vi "ReadINI.vi"(8 "error in (no error)":errorcluster) -> (0 "error out":errorcluster, 2 "FileNotFound/Corrupted?":bool, 3 "value":T1={"ClientTimeout (s)"=30, "LogPath"=path "", "CriticalErrors"=[], "OracleData"={"DBname"="", "User"="", "Password"=""}})   [LabVIEW 2017, in "Server.lvlib"]
doc: "Reads the INI-File and decodes the XML-String to ServerINI.ctl-Cluster. If File not found or File content doesnt fit to the ctl it outputs a bool."
uses:
  Server.lvlib
  TypeDefs/ServerINI.ctl
  SubLibs/Oracle/OracleData.ctl
  SubLibs/Oracle/Oracle.lvlib
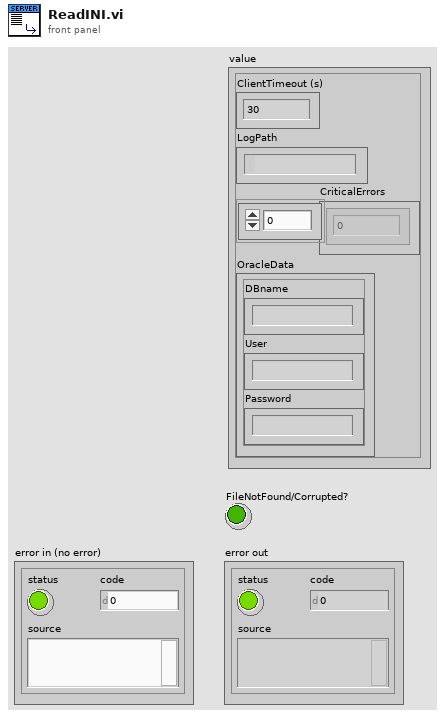
[diagram p1: front panel]
types:
  T1 = typedef "Server.lvlib/ServerINI.ctl" = cluster{"ClientTimeout (s)":u32, "LogPath":path, "CriticalErrors":i32[], "OracleData":T2}
  T2 = typedef "Server.lvlib/Oracle.lvlib/OracleData.ctl" = cluster{"DBname":string, "User":string, "Password":string}
  T3 = enum16{"open", "replace", "create", "open or create", "replace or create", "replace or create with confirmation"}
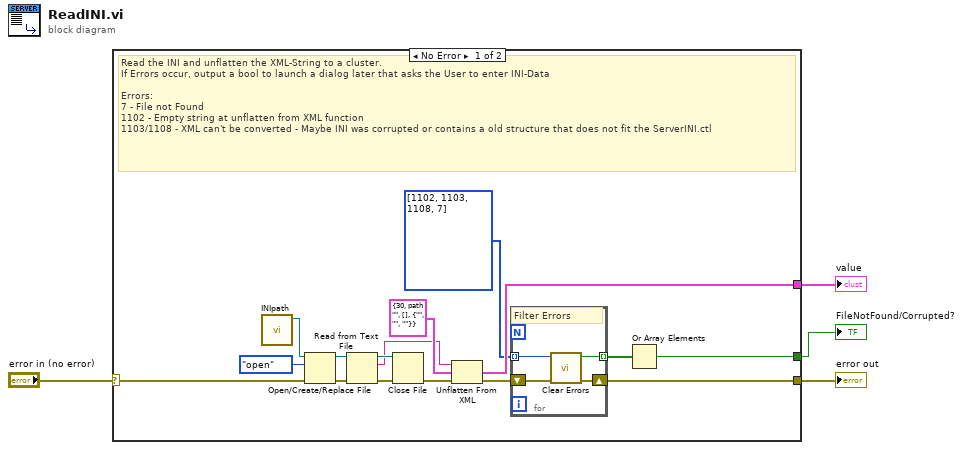
[diagram p0: block diagram]
diagram:
  n1 = case shown="No Error" "error in (no error)" {
    selector: "error in (no error)" -> [w11 w25]
    tunnel: [w7 w25] -> w4
    tunnel: [w18 _] -> w3
    tunnel: [w5 _] -> w1
    frame No Error {
      # "Read the INI and unflatten the XML-String to a cluster.\nIf Errors occur, output a bool to launch a dialog later that asks the User to enter INI-Data\n\nErrors:\n7 - File not Found\n1102 - Empty string at unflatten from XML function\n1103/1108 - XML can't be converted - Maybe INI was corrupted or contains a old structure that does not fit the ServerINI.ctl"
      n2 = call "INIpath.vi"() -> ("appended path"=w20:path)  [unwired: 11 in]
      n3 = Open/Create/Replace File(file path (use dialog)=w20, error in=w11, operation (0:open)=T3."open") -> (refnum out=w16:refnum<file>, error out=w13:errorcluster)  [unwired: 3 in, 1 out]
      n4 = Read from Text File(file (use dialog)=w16, error in=w13) -> (refnum out=w17:refnum<file>, text=w6:string, error out=w14:errorcluster)  [unwired: 2 in, 1 out]
      n5 = Close File(refnum=w17, error in=w14) -> (error out=w15:errorcluster)  [unwired: 1 out]
      n6 = Unflatten From XML(xml string=w6, type=T1 {"ClientTimeout (s)"=30, "LogPath"=path "", "CriticalErrors"=[], "OracleData"={"DBname"="", "User"="", "Password"=""}} ("ServerINI"), error in (no error)=w15) -> (value=w18:T1, error out=w8:errorcluster)
      n7 = for {
        tunnel: [w24] -> w10 mode=indexing
        tunnel: i32[] [1102, 1103, 1108, 7] ("specific error code to clear (0: all)") -> [w23] mode=indexing
        shift-right: [w21] -> w7
        shift-left: w8 -> [w22]
        # "Filter Errors"
        n8 = call <vilib>:"Clear Errors.vi"("error in (no error)"=w22, "specific error code to clear (0: all)"=w23) -> ("error out"=w21:errorcluster, "specific error cleared?"=w24:bool)  [unwired: 4 in]
      }
      n9 = Or Array Elements(Boolean array=w10) -> (logical OR=w5:bool)
    }
    frame Error {
    }
  }
  "value" <- w3
  "error out" <- w4
  "FileNotFound/Corrupted?" <- w1
